vi "plantita.vi"() -> ()   [LabVIEW 2014]
uses:
  <vilib>/addons/control/pid/NI_PID_pid.lvlib
  <vilib>/addons/control/pid/pid.llb/PID (DBL).vi
  state.ctl
  <vilib>/DAQmx/write.llb/DAQmx Write (Analog DBL 1Chan 1Samp).vi
  calcDoseorGetGraph.ctl
  Manual or Auto.ctl
  setpoints.ctl
panel:
  out "Fitting Params":cluster{dbl[], "Best Linear Fit":dbl[]}[](graph)
  in  "setpoints":T1={"target clarified turbidity (NTU)"=0.3, "flocculator volume (L)"=0.0, "clarifier volume (L)"=0.0, "dose updates per HRT"=100} {"target clarified turbidity (NTU)" min=0.1 max=5.0 step=0.01; "dose updates per HRT" min=1 max=1000 step=1}
  out "stopping":bool
  in  "Coagulant":T2
  out "data labels":string[](array[string])
  in  "Backwash control":T2
  in  "Smoothed":bool
  in  "Sludge control":bool
  in  "Sludge valve [V]":dbl(slide)=1.5 scale=0.0..5.0
  in  "Coagulant  [mg/L]":dbl(slide) scale=0.0..50.0
  in  "Main valve [V]":dbl(slide)=2.5 scale=0.0..5.0
  in  "Flow control":bool
  out "Main valve":dbl(graph)
  in  "Shut Down":bool
  out "flocculated [NTU]":dbl
  out "Save File Path 2":path=path "C:/1.tdms"
  out "filtered [NTU]":dbl
  out "settled [NTU]":dbl
  out "raw water [NTU]":dbl
  in  "Ripen time [s]":dbl=600.0
  in  "min filtration time [s]":dbl=600.0
  out "Last backwash":timestamp
  in  "Filtered quality target [NTU]":dbl=0.3
  out "Coagulant [mg Al/L]":dbl(graph)
  out "Turbidities":dynamicdata(graph)
  out "UV 254":dbl(graph)
  in  "Sludge flow target [L/min]":dbl=0.84
  in  "Sludge PID":T3={"proportional gain (Kc)"=0.07, "integral time (Ti, min)"=1.0, "derivative time (Td, min)"=0.01} {"derivative time (Td, min)" format="%.3f"; "integral time (Ti, min)" format="%.3f"; "proportional gain (Kc)" format="%.3f"}
  in  "Plant Flow PID":T3={"proportional gain (Kc)"=0.05, "integral time (Ti, min)"=1.0, "derivative time (Td, min)"=0.01} {"derivative time (Td, min)" format="%.3f"; "integral time (Ti, min)" format="%.3f"; "proportional gain (Kc)" format="%.3f"}
  in  "Main flow [L/min]":dbl=30.0
  out "Filter head loss":dbl
  out "Water flow [L/s]":dbl
  out "Sludge flow value":dbl
  in  "backwash [ON/OFF]":bool
  out "Sludge valve":dbl(graph)
  out "Sludge flow meter":dbl(graph)
  out "Filter head loss":dbl(graph)
  out "Main flow meter":dbl(graph)
  in  "DAQ data interval [s]":dbl=1.0
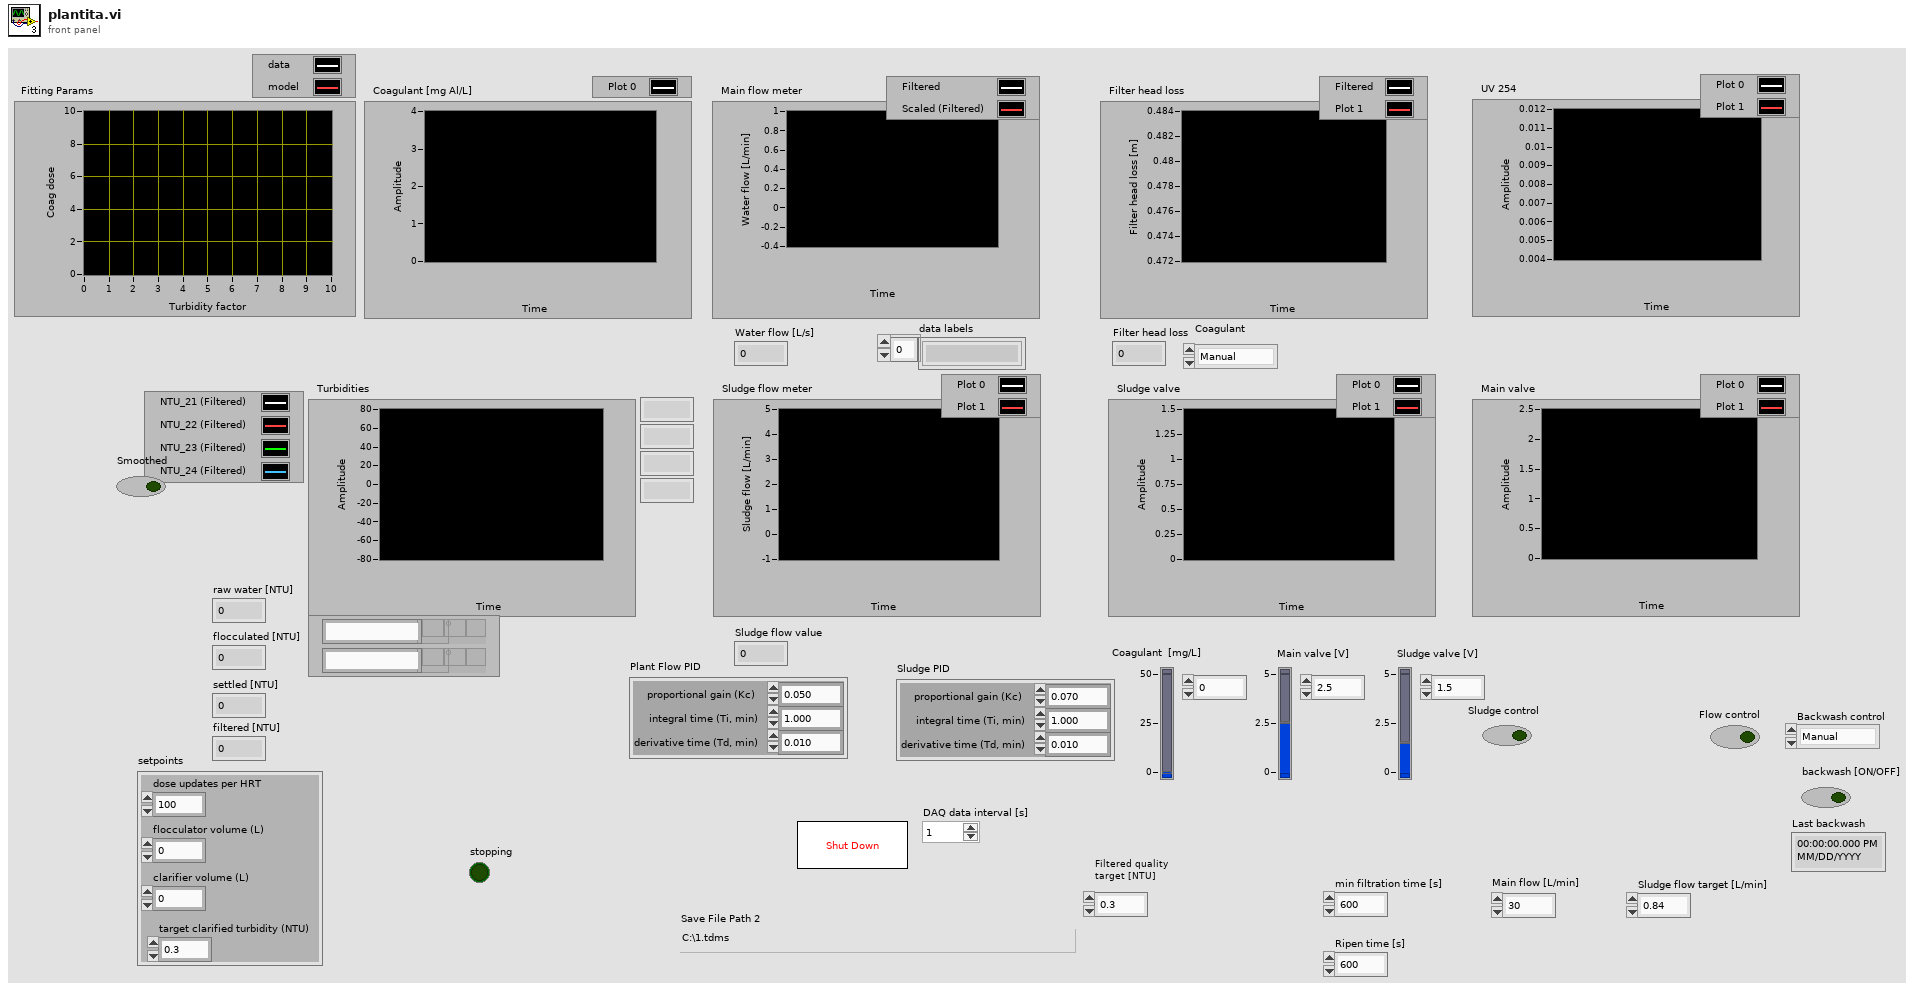
[diagram p1: front panel]
types:
  T1 = typedef "setpoints.ctl" = cluster{"target clarified turbidity (NTU)":dbl, "flocculator volume (L)":dbl, "clarifier volume (L)":dbl, "dose updates per HRT":u32}
  T2 = typedef "Manual or Auto.ctl" = enum16{"Manual", "Automatic"}
  T3 = cluster{"proportional gain (Kc)":dbl, "integral time (Ti, min)":dbl, "derivative time (Td, min)":dbl}
  T4 = enum16{"open", "open or create", "create or replace", "create", "open (read-only)"}
  T5 = typedef "state.ctl" = enum16{"Initialize", "Change setpoints", "Process data", "Close"}
  T6 = typedef "calcDoseorGetGraph.ctl" = enum16{"calculate dose", "read graph"}
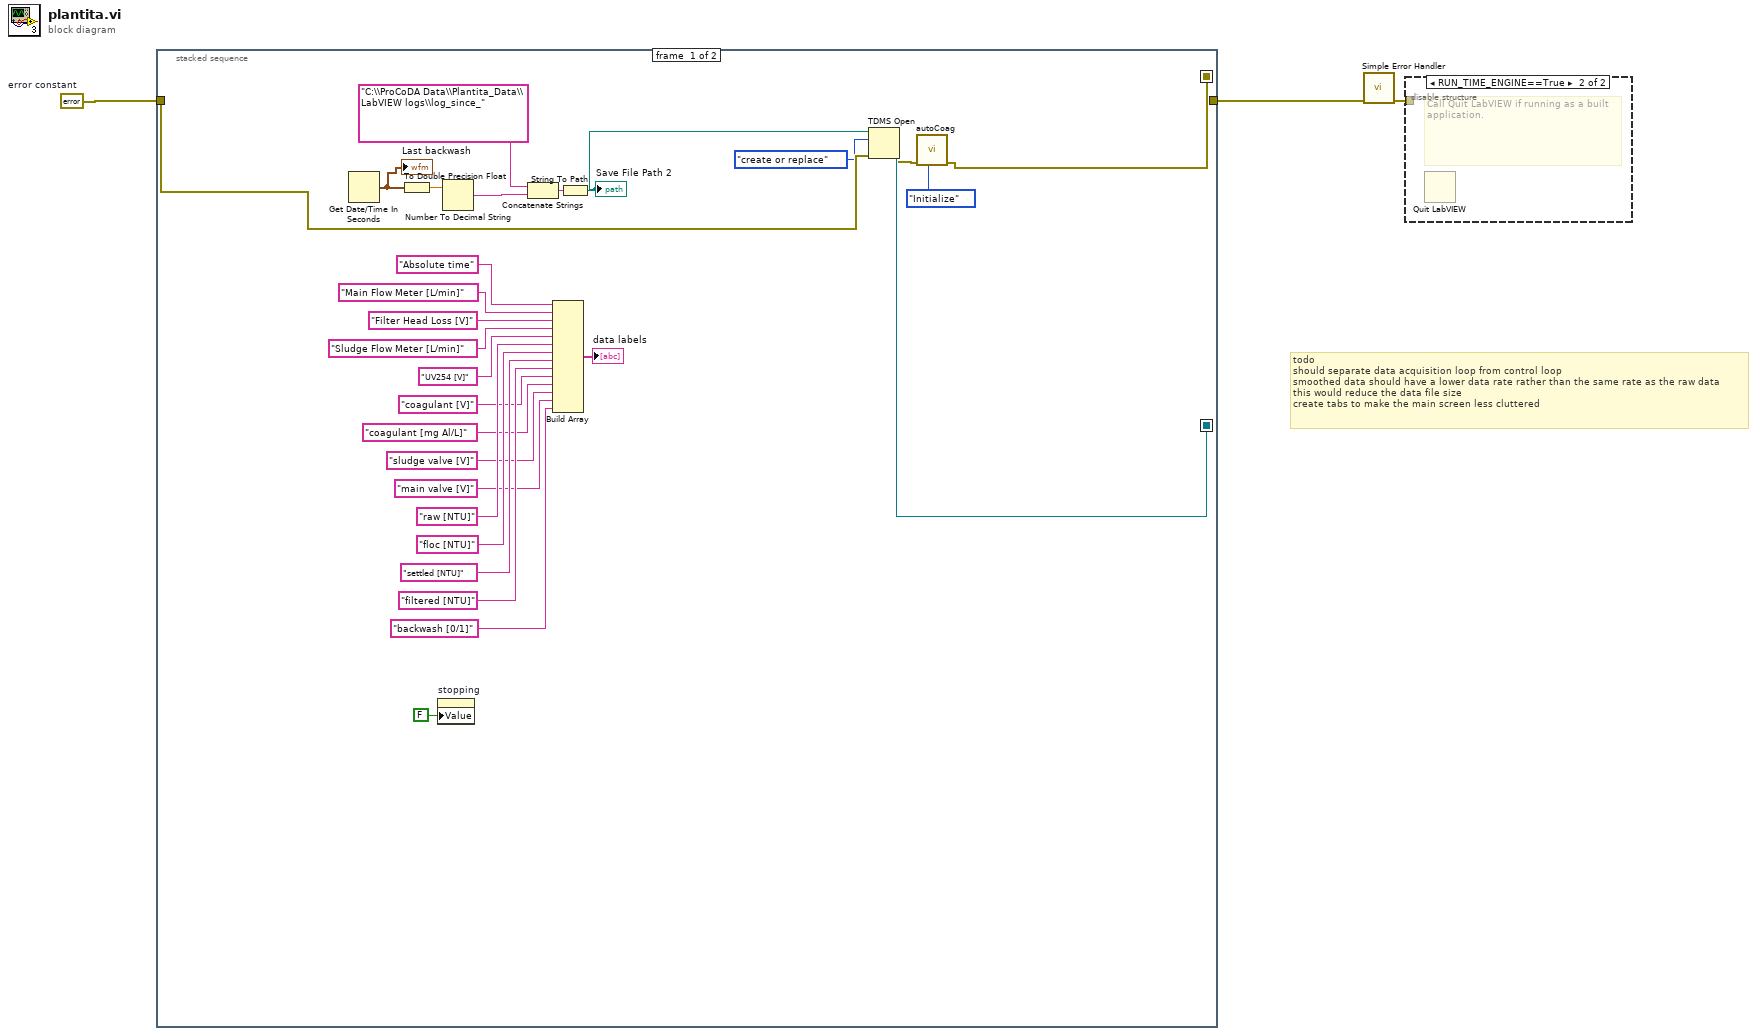
[diagram p0: block diagram]
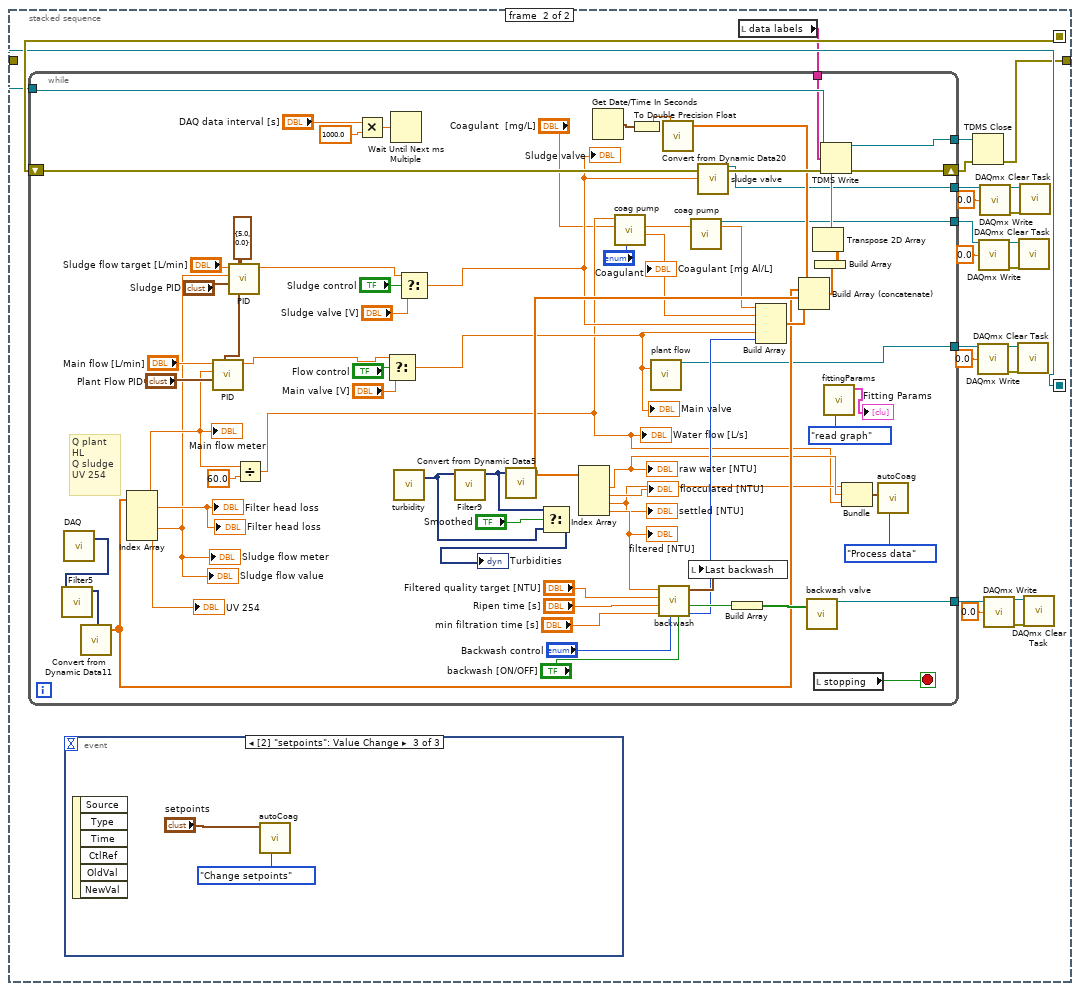
[diagram p2: hidden frame]
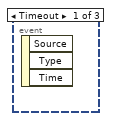
[diagram p3: hidden frame]
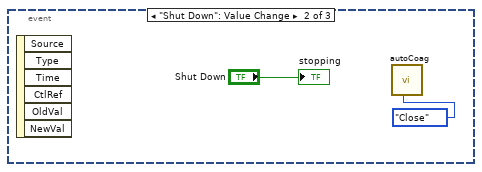
[diagram p4: hidden frame]
diagram:
  w3 = errorcluster {"status"=FALSE, "code"=0, "source"=""}  # error constant
  # "todo\nshould separate data acquisition loop from control loop\nsmoothed data should have a lower data rate rather than the same rate as the raw data\nthis would reduce the data file size\ncreate tabs to make the main screen less cluttered"
  n1 = stacked-sequence {
    seq-local: [w31 _] -> [_ w52]
    seq-local: [w13 _] -> [_ w53]
    tunnel: w3 -> [w12 _]
    tunnel: [_ w48] -> w2
    frame #0 {
      n2 = Get Date/Time In Seconds() -> (seconds since 1Jan1904=w8:timestamp)
      "Last backwash" <- w8
      n3 = To Double Precision Float(number=w8) -> (double precision float=w11:dbl)
      n4 = property on="stopping" class="Bool (strict)"("Value"=FALSE ("stopping")) -> ()  [unwired: 2 in, 2 out]
      n5 = Number To Decimal String(number=w11) -> (decimal integer string=w10:string)  [unwired: 1 in]
      n6 = Concatenate Strings("C:\\ProCoDA Data\\Plantita_Data\\LabVIEW logs\\log_since_", w10) -> (w9:string)
      n7 = Build Array("Absolute time", "Main Flow Meter [L/min]", "Filter Head Loss [V]", "Sludge Flow Meter [L/min]", "UV254 [V]" ("element"), "raw [NTU]", "floc [NTU]", "settled [NTU]", "filtered [NTU]" ("element"), "coagulant [V]" ("element"), "coagulant [mg Al/L]" ("element"), "sludge valve [V]" ("element"), "main valve [V]" ("element"), "backwash [0/1]" ("element")) -> (→"data labels":string[])
      n8 = String To Path(string=w9) -> (path=w5:path)
      "Save File Path 2" <- w5
      n9 = TDMS Open(8:w12, 10:T4."create or replace" ("operation (0:open)"), 11:w5) -> (0:w14:errorcluster, 3:w31:refnum<k34>)  [unwired: 4 in]
      n10 = call "autoCoag.vi"("Enum"=state."Initialize", "error in (no error)"=w14) -> ("error out"=w13:errorcluster)  [unwired: 8 in, 1 out]
    }
    frame #1 {
      n11 = event shown="[2] \"setpoints\": Value Change" {
        selector: _ -> [_ _ _]
        dyn-events: _ -> [_ _ _]
        timeout: _ -> [_ _ _]
        event Timeout {
          n12 = event-data() -> ()  [unwired: 1 in, 3 out]
        }
        event "Shut Down": Value Change {
          n13 = event-data() -> ()  [unwired: 1 in, 6 out]
          n14 = call "autoCoag.vi"("Enum"=state."Close") -> ()  [unwired: 9 in, 2 out]
          "stopping" <- "Shut Down"
        }
        event Value Change {
          n15 = event-data() -> ()  [unwired: 1 in, 6 out]
          n16 = call "autoCoag.vi"("Enum"=state."Change setpoints", "setpoints"="setpoints") -> ()  [unwired: 8 in, 2 out]
        }
      }
      n17 = local read "data labels"() -> (w49:string[])
      n18 = while {
        shift-right: [w121] -> w51
        shift-left: w53 -> [w123]
        tunnel: w52 -> [w122]
        tunnel: [w120] -> w50
        tunnel: w49 -> [w77]
        tunnel: [w67] -> w47
        tunnel: [w66] -> w41
        tunnel: [w65] -> w37
        tunnel: [w60] -> w33
        stop <- w110 stop-if-true
        w78 = cluster{"output high":dbl, "output low":dbl} {"output high"=5.0, "output low"=0.0} ("output range")
        # "Q plant\nHL\nQ sludge\nUV 254"
        n19 = call "DAQ"() -> ("data"=w96:dynamicdata)  [unwired: 17 in, 2 out]
        n20 = call "Filter5"("Signal"=w96) -> ("Filtered Signal"=w94:dynamicdata)  [unwired: 9 in, 1 out]
        n21 = call "Convert from Dynamic Data11"("Dynamic Data Type"=w94) -> ("Array"=w85:dbl[])  [unwired: 3 in]
        n22 = Index Array(array=w85) -> (element #1=w84:dbl, element #2=→"Filter head loss" →"Filter head loss":dbl, element #3=w82:dbl, element #4=→"UV 254":dbl)  [unwired: 4 in]
        "Main flow meter" <- w84
        "Sludge flow meter" <- w82
        "Sludge flow value" <- w82
        n23 = call-poly <vilib>:"PID.vi"("output range"=w78, "PID gains"="Plant Flow PID", "process variable"=w84, "setpoint"="Main flow [L/min]") -> ("output"=w111:dbl)  [unwired: 6 in, 1 out]
        n24 = call-poly <vilib>:"PID.vi"("output range"=w78, "PID gains"="Sludge PID", "process variable"=w82, "setpoint"="Sludge flow target [L/min]") -> ("output"=w80:dbl)  [unwired: 6 in, 1 out]
        n25 = Divide(x=w84, y=60.0) -> (x/y=w73:dbl)
        "Water flow [L/s]" <- w73
        n26 = Multiply(x="DAQ data interval [s]", y=1000.0) -> (x*y=w125:dbl)
        n27 = Select(t=w111, s="Flow control", f="Main valve [V]") -> (s? t:f=w91:dbl)
        "Main valve" <- w91
        n28 = Wait Until Next ms Multiple(millisecond multiple=w125) -> ()  [unwired: 1 out]
        n29 = call "turbidity"() -> ("data"=w107:dynamicdata)  [unwired: 17 in, 2 out]
        n30 = Select(t=w80, s="Sludge control", f="Sludge valve [V]") -> (s? t:f=w92:dbl)
        "Sludge valve" <- w92
        n31 = call "Filter9"("Signal"=w107) -> ("Filtered Signal"=w95:dynamicdata)  [unwired: 9 in, 1 out]
        n32 = call "Convert from Dynamic Data5"("Dynamic Data Type"=w95) -> ("Array"=w93:dbl[])  [unwired: 3 in]
        n33 = Select(t=w95, s="Smoothed", f=w107) -> (s? t:f=→"Turbidities":dynamicdata)
        n34 = Index Array(array=w93) -> (element #1=w75:dbl, element #2=→"flocculated [NTU]":dbl, element #3=w74:dbl, element #4=w97:dbl)  [unwired: 4 in]
        "raw water [NTU]" <- w75
        "settled [NTU]" <- w74
        "filtered [NTU]" <- w97
        n35 = Get Date/Time In Seconds() -> (seconds since 1Jan1904=w116:timestamp)
        n36 = call "coag pump.vi"("Coagulant control"="Coagulant", "coagulant dose [mg/L]"="Coagulant  [mg/L]", "plant flow [L/s]"=w73) -> ("coag dose [mg/L]"=w70:dbl, "pump [V]"=w79:dbl)  [unwired: 6 in, 1 out]
        "Coagulant [mg Al/L]" <- w70
        n37 = To Double Precision Float(number=w116) -> (double precision float=w115:dbl)
        n38 = call "plant flow"("data"=w91) -> ("task out"=w60:refnum<k21>)  [unwired: 17 in, 1 out]
        n39 = call "backwash.vi"("Manual override"="backwash [ON/OFF]", "Backwash control"="Backwash control", "min filtration time [s]"="min filtration time [s]", "Ripen time [s]"="Ripen time [s]", "Filtered quality target [NTU]"="Filtered quality target [NTU]", "Filtered Turbidity"=w97) -> (0:"backwashing?"=w90:i16, 1:"backwashing?"=w104:bool, "last backwash"=w98:timestamp)  [unwired: 3 in]
        n40 = call "Convert from Dynamic Data20"("Dynamic Data Type"=w115) -> ("Array"=w112:dbl[])  [unwired: 3 in]
        n41 = local write "Last backwash"(w98) -> ()
        n42 = call "coag pump"("data"=w79) -> ("task out"=w66:refnum<k21>)  [unwired: 17 in, 1 out]
        n43 = call "sludge valve"("data"=w92) -> ("task out"=w67:refnum<k21>)  [unwired: 17 in, 1 out]
        n44 = Build Array(w104) -> (w105:bool[])
        n45 = Build Array(w79, w70, w92, w91, w90) -> (w89:dbl[])
        n46 = Build Array (concatenate)(w112, w85, w93, w89) -> (w88:dbl[])
        n47 = call "backwash valve"("data"=w105) -> ("task out"=w65:refnum<k21>)  [unwired: 17 in, 1 out]
        n48 = local read "stopping"() -> (w110:bool)
        n49 = Build Array(w88) -> (w87:dbl[][])
        n50 = Transpose 2D Array(2D array=w87) -> (transposed array=w86:dbl[][])
        n51 = TDMS Write(0:w122, 7:w77, 9:w86, 11:w123) -> (4:w120:refnum<k34>, 15:w121:errorcluster)  [unwired: 2 in, 2 out]
        n52 = call "fittingParams.vi"("read/write"=calcDoseorGetGraph."read graph") -> ("Fitting Params"=→"Fitting Params":cluster{dbl[], "Best Linear Fit":dbl[]}[])  [unwired: 6 in, 3 out]
        n53 = Bundle(w74, w75, w73) -> (w72:cluster{dbl, dbl, dbl})  [unwired: 1 in]
        n54 = call "autoCoag.vi"("Enum"=state."Process data", "data input"=w72) -> ()  [unwired: 8 in, 2 out]
      }
      n55 = TDMS Close(8:w51, 11:w50) -> (0:w48:errorcluster)  [unwired: 1 out]
      n56 = call-poly <vilib>:"DAQmx Write.vi"("task/channels in"=w33, "data"=0.0) -> ("task out"=w32:refnum<k21>, "error out"=w35:errorcluster)  [unwired: 11 in, 1 out]
      n57 = call-poly <vilib>:"DAQmx Write.vi"("task/channels in"=w41, "data"=0.0) -> ("task out"=w40:refnum<k21>, "error out"=w42:errorcluster)  [unwired: 11 in, 1 out]
      n58 = call-poly <vilib>:"DAQmx Write.vi"("task/channels in"=w47, "data"=0.0) -> ("task out"=w46:refnum<k21>, "error out"=w45:errorcluster)  [unwired: 11 in, 1 out]
      n59 = call-poly <vilib>:"DAQmx Write.vi"("task/channels in"=w37, "data"=0.0) -> ("task out"=w36:refnum<k21>, "error out"=w39:errorcluster)  [unwired: 11 in, 1 out]
      n60 = call <vilib>:"DAQmx Clear Task.vi"("task in"=w32, "error in"=w35) -> ()  [unwired: 13 in, 1 out]
      n61 = call <vilib>:"DAQmx Clear Task.vi"("task in"=w40, "error in"=w42) -> ()  [unwired: 13 in, 1 out]
      n62 = call <vilib>:"DAQmx Clear Task.vi"("task in"=w46, "error in"=w45) -> ()  [unwired: 13 in, 1 out]
      n63 = call <vilib>:"DAQmx Clear Task.vi"("task in"=w36, "error in"=w39) -> ()  [unwired: 13 in, 1 out]
    }
  }
  n64 = call <vilib>:"Simple Error Handler.vi"("error in (no error)"=w2) -> ("error out"=w1:errorcluster)  [unwired: 4 in, 4 out]
  n65 = disable-structure shown="RUN_TIME_ENGINE==True" {
    disable-tunnel: w1 -> [_ _]
    frame condition #0 (active) {
    }
    frame condition #1 {
      # "Call Quit LabVIEW if running as a built application."
      n66 = Quit LabVIEW() -> ()  [unwired: 1 in]
    }
  }
